vi "Measure DC Voltage.vi"(7 "ValBufferSize":i32=2048, 8 "error in (no error)":errorcluster {"code" format="%.0x"}, 9 "MaxTimeMilliseconds":i32 format="%.0g", 10 "ChannelList":string, 11 "instrument handle":refnum<k15>) -> (0 "error out":errorcluster {"code" format="%.0x"}, 1 "ValActualSize":i32, 2 "Val":dbl[](array[numeric]) format="%.2p", 3 "instrument handle out":refnum<k15>)   [LabVIEW 2020, in "Keysight DAQ970.lvlib"]
doc: "Configure the specified channels for DC Voltage autorange measurements, immediately sweep through the scan list once, and read the measured data. Note: This command redefines the scan list."
uses:
  Keysight DAQ970.lvlib
  KtDAQ970.dll
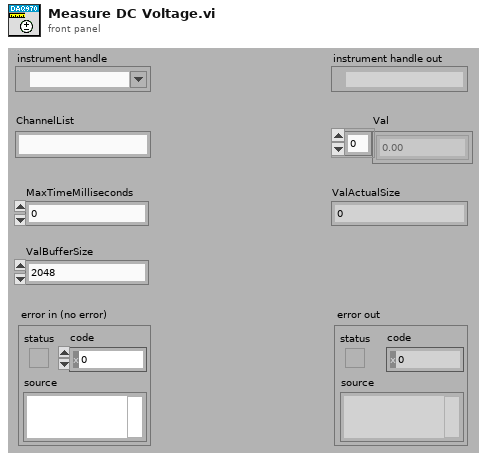
[diagram p1: front panel]
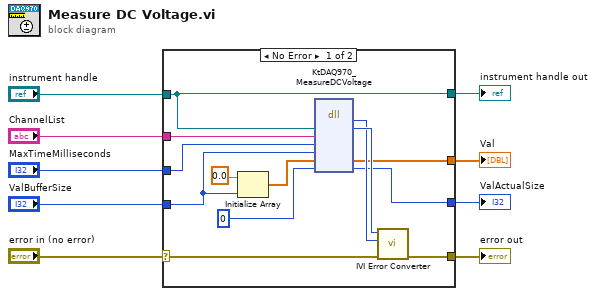
[diagram p0: block diagram]
diagram:
  n1 = case shown="No Error" "error in (no error)" {
    selector: "error in (no error)" -> [w20 w24]
    tunnel: [w19 w24] -> w9
    tunnel: "instrument handle" -> [w11 w23]
    tunnel: "ChannelList" -> [w18 _]
    tunnel: "MaxTimeMilliseconds" -> [w17 _]
    tunnel: "ValBufferSize" -> [w10 _]
    tunnel: [w14 _] -> w3
    tunnel: [w12 _] -> w2
    tunnel: [w11 w23] -> w1
    frame No Error {
      n2 = Initialize Array(0.0 ("element"), w10) -> (w16:dbl[])
      n3 = dll-call lib="KtDAQ970**.dll" fn="KtDAQ970_MeasureDCVoltage"("Vi"=w11, "ChannelList"=w18, "MaxTimeMilliseconds"=w17, "ValBufferSize"=w10, "Val"=w16, "ValActualSize"=0) -> ("return type"=w21:i32, "Vi"=w22:u32, "Val"=w14:dbl[], "ValActualSize"=w12:i32)  [unwired: 6 in, 2 out]
      n4 = call "IVI Error Converter.vi"("error in (no error)"=w20, "IVI error code (0)"=w21, "instrument handle"=w22) -> ("error out"=w19:errorcluster)  [unwired: 7 in, 1 out]
    }
    frame Error {
    }
  }
  "error out" <- w9
  "instrument handle out" <- w1
  "Val" <- w3
  "ValActualSize" <- w2
